vi "TempMeas.vi"() -> ()   [LabVIEW 2017]
uses:
  Control 1.ctl
  <vilib>/DAQmx/read.llb/DAQmx Read (Analog 1D Wfm NChan 1Samp).vi
  <vilib>/DAQmx/miscellaneous.llb/DAQmx Fill In Error Info.vi
panel:
  out "Ścieżka zapisu":path
  out "Waveform Chart - Dark":waveform(dbl)[](graph)
  in  "Refresh Square":bool
  in  "Save Square":bool
  in  "Pause Square":bool
  in  "Start Square":bool
  in  "wybor wykresu":T1
  in  "stop":bool
  out "wsk startu":bool
  in  "Enum":T2(ring)
  in  "DAQmx Task Name":refnum<k21>="temperature_task"
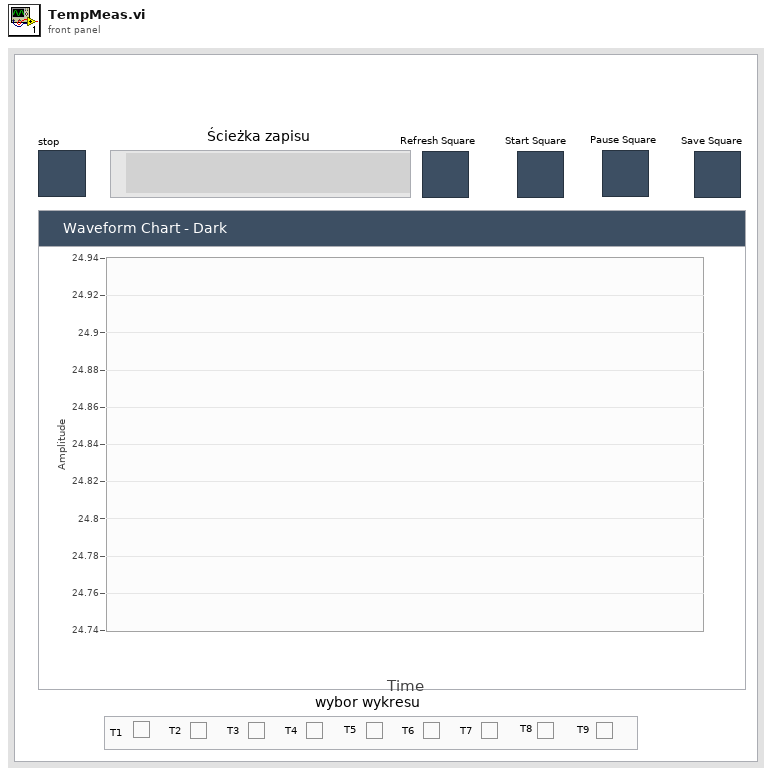
[diagram p1: front panel]
types:
  T1 = typedef "Control 1.ctl" = cluster{"T1":bool, "T2":bool, "T3":bool, "T4":bool, "T6":bool, "T5":bool, "T7":bool, "T8":bool, "T9":bool}
  T2 = enum16{"init", "start", "pause", "save", "exit", "refresh", "wait for event"}
  T3 = enum8{"Enabled", "Disabled", "Disabled and Grayed Out"}
  T4 = enum16{"open", "open or create", "create or replace", "create", "open (read-only)"}
  T5 = enum16{"init", "start", "pause", "save", "exit", "refresh"}
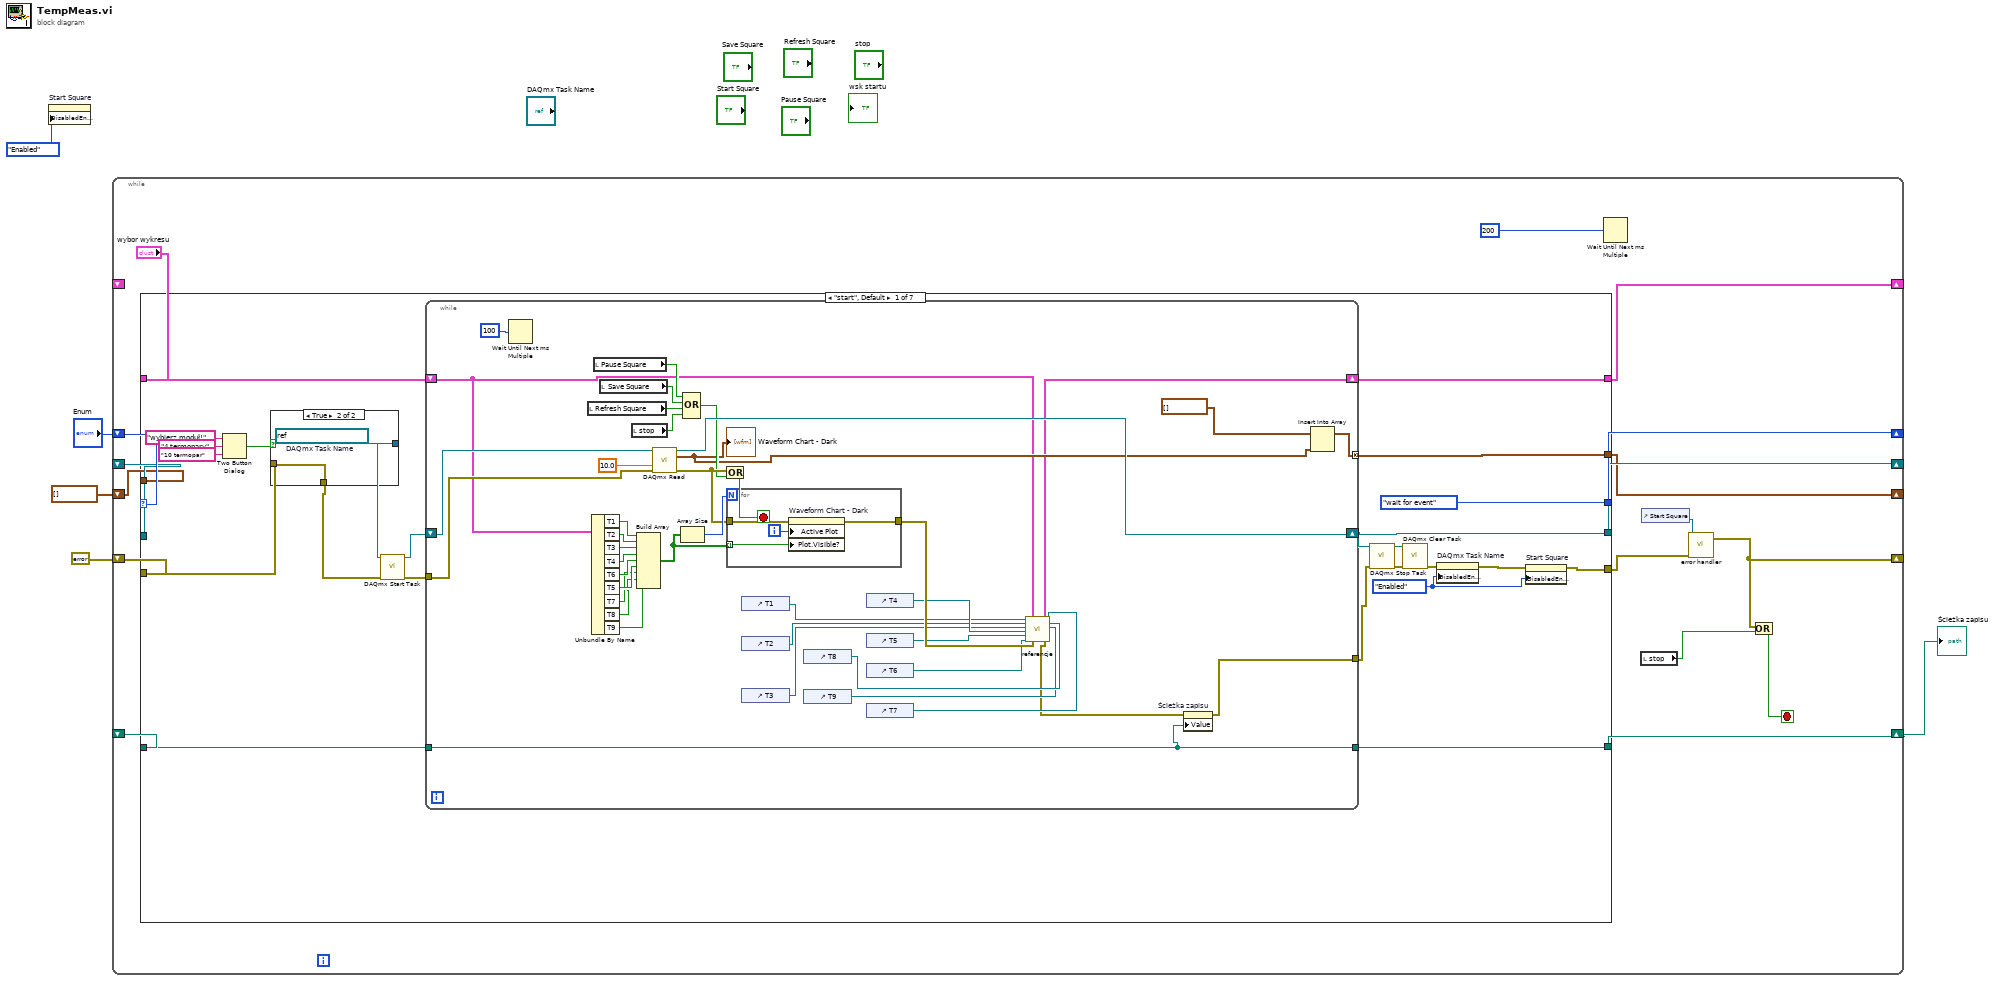
[diagram p0: block diagram]
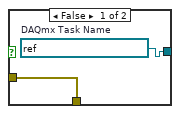
[diagram p2: hidden frame]
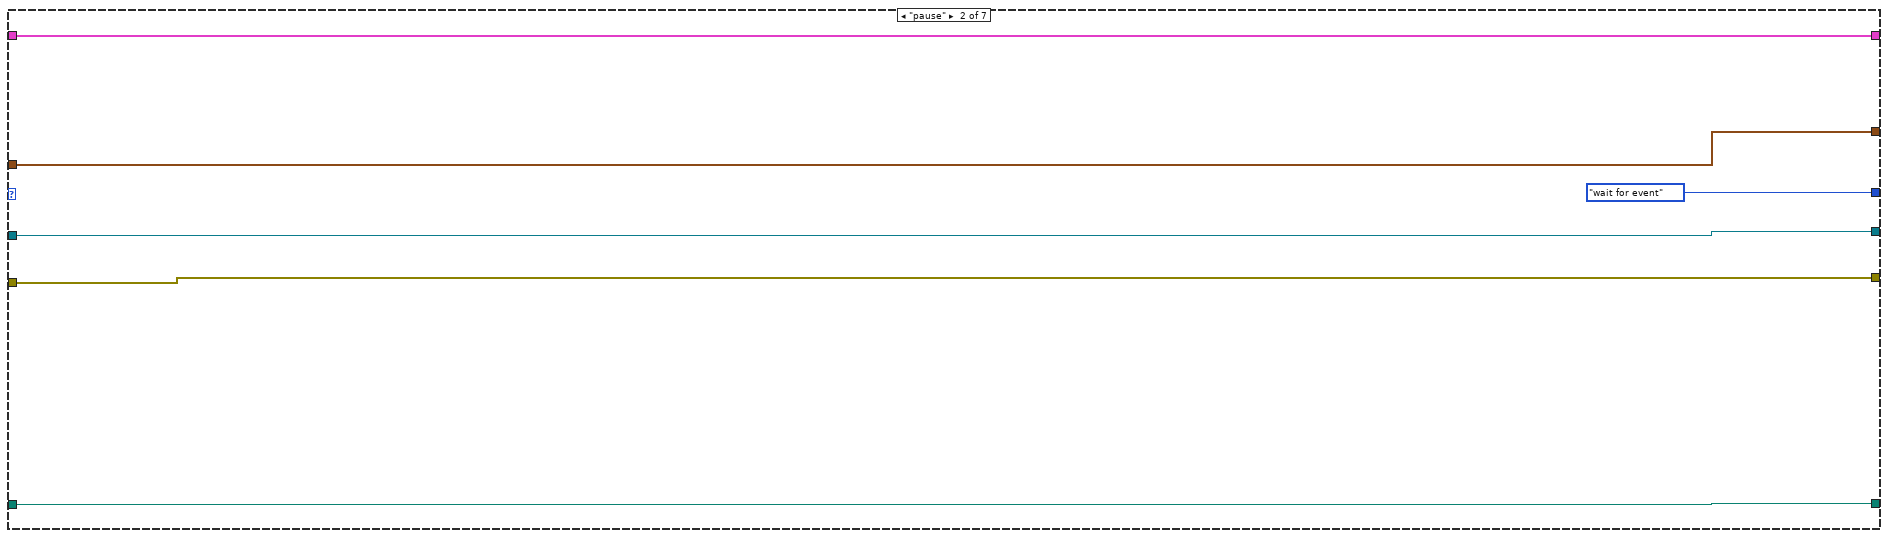
[diagram p3: hidden frame]
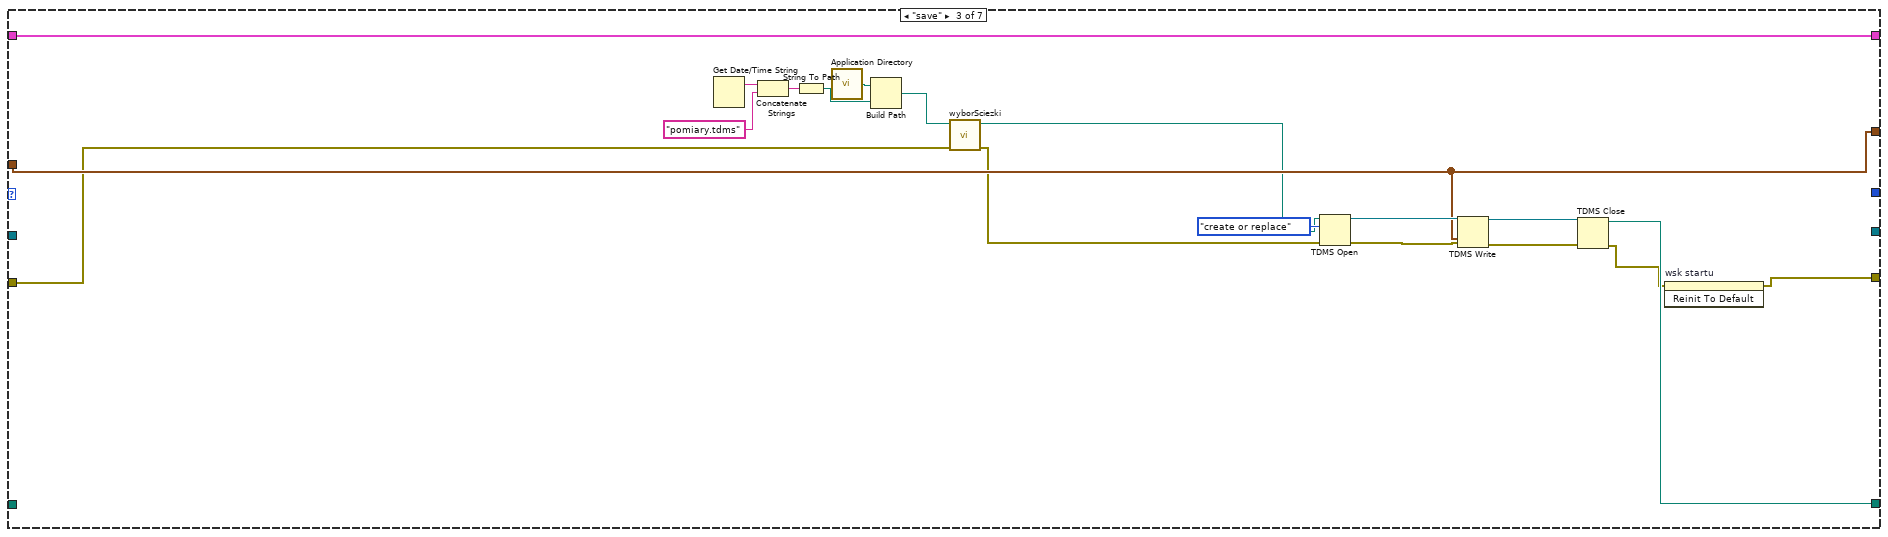
[diagram p4: hidden frame]
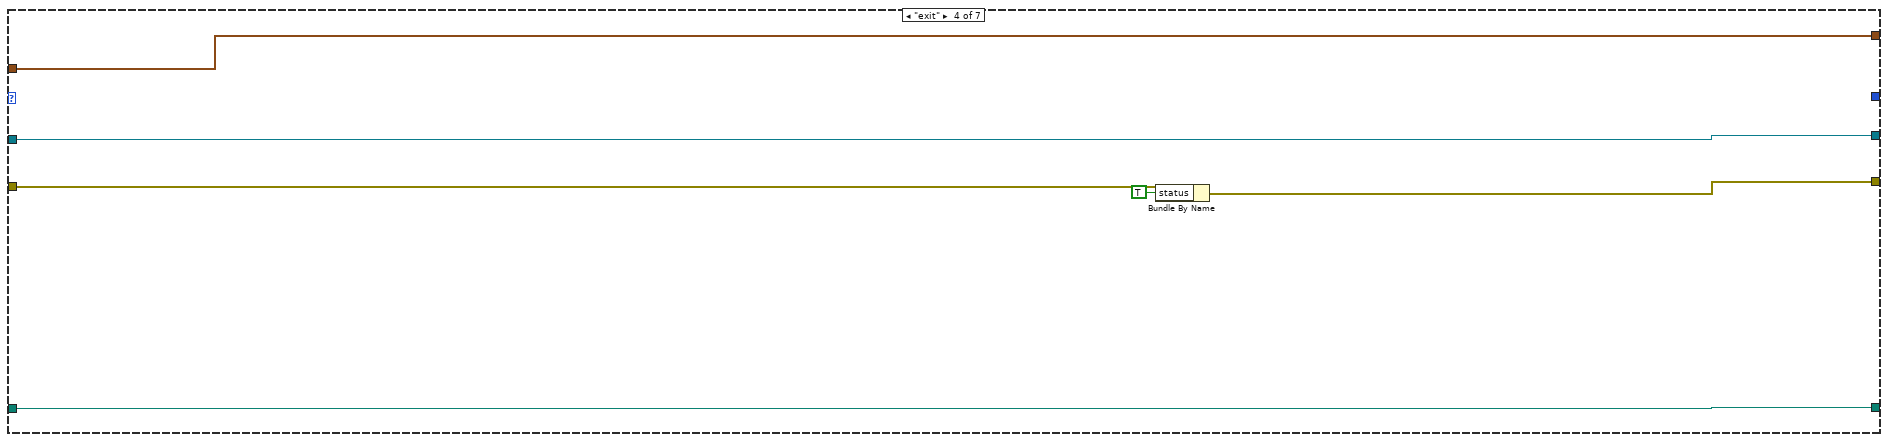
[diagram p5: hidden frame]
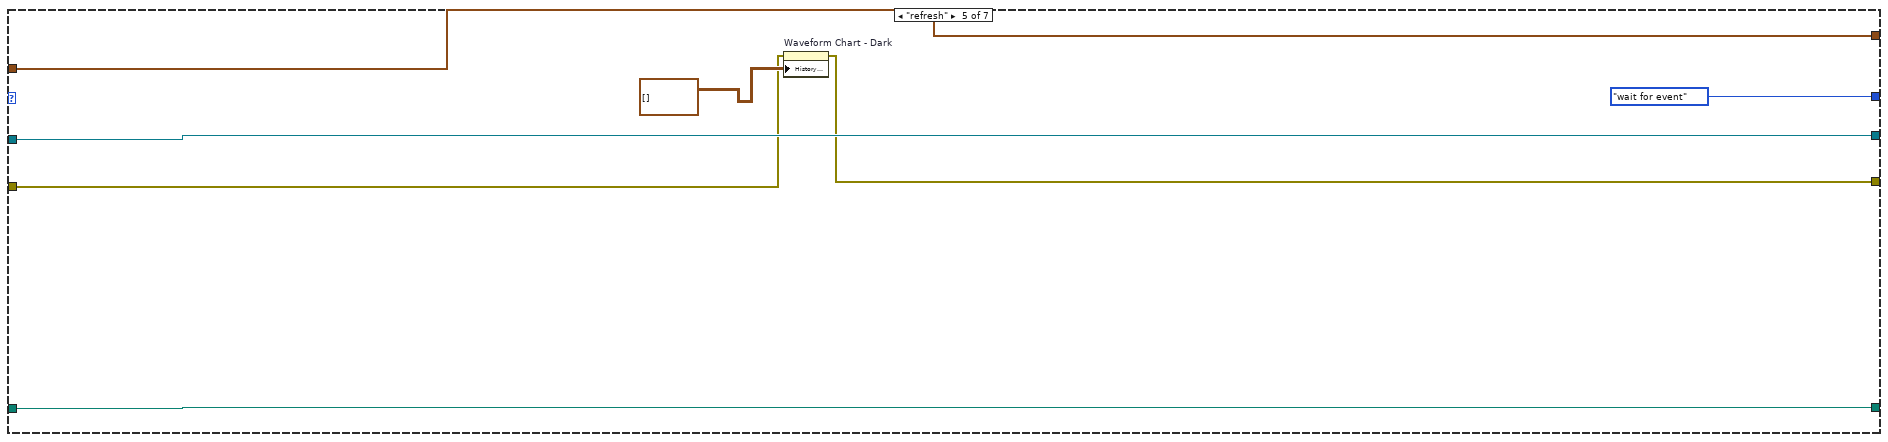
[diagram p6: hidden frame]
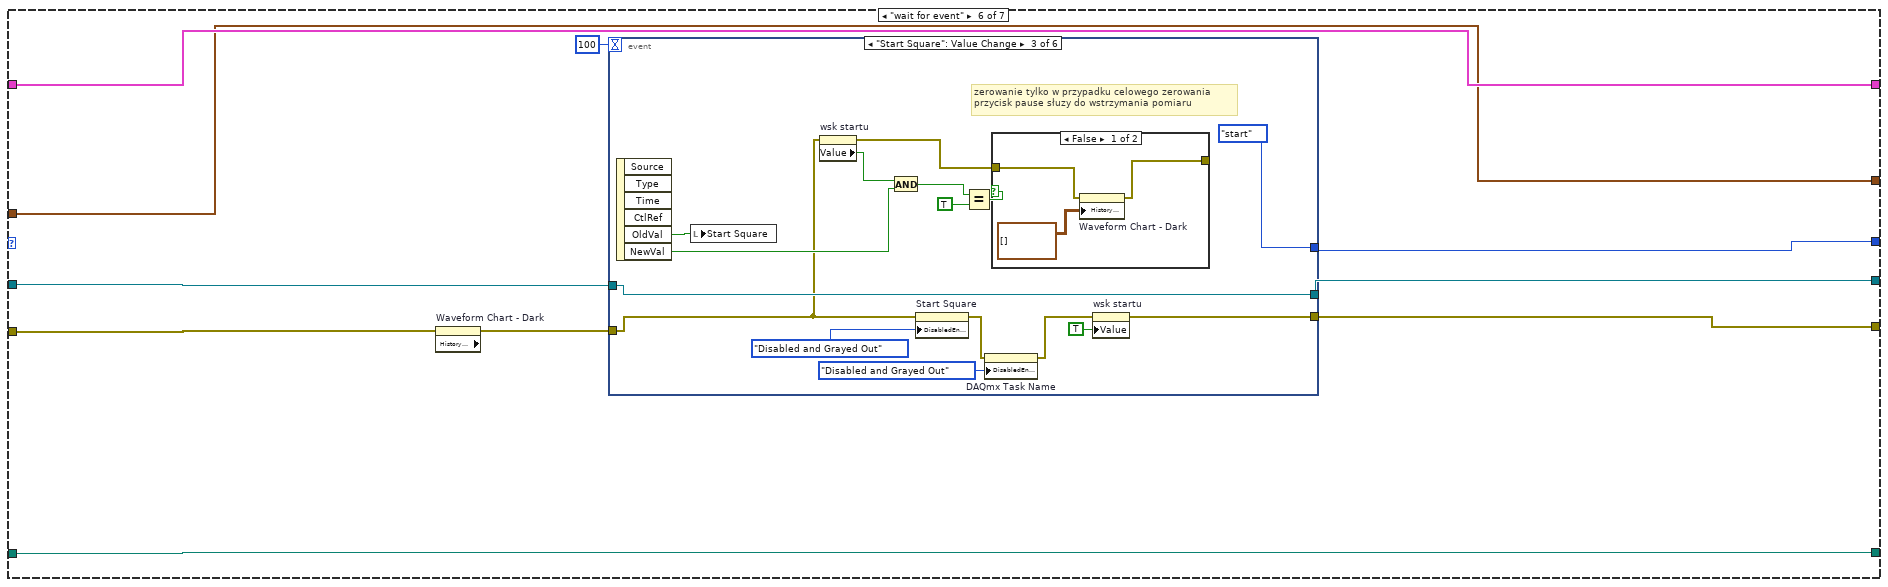
[diagram p7: hidden frame]
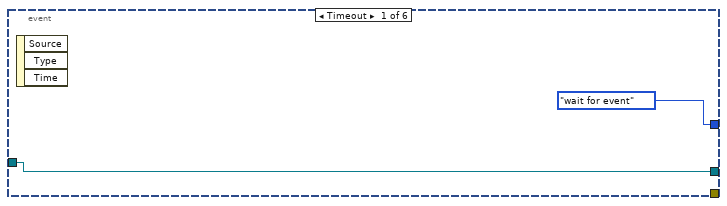
[diagram p8: hidden frame]
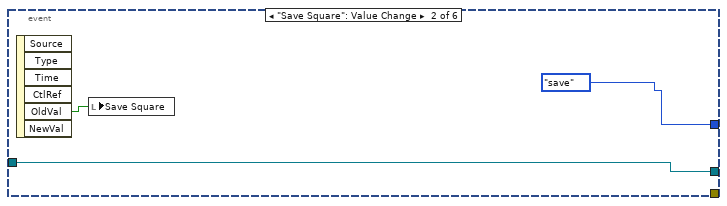
[diagram p9: hidden frame]
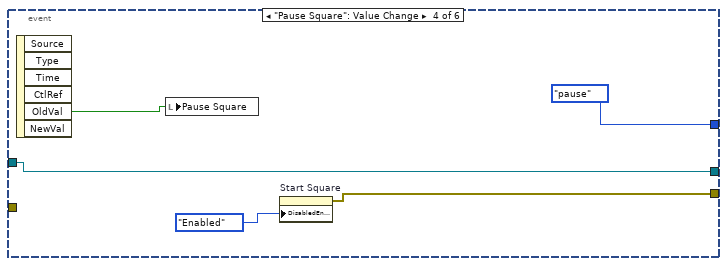
[diagram p11: hidden frame]
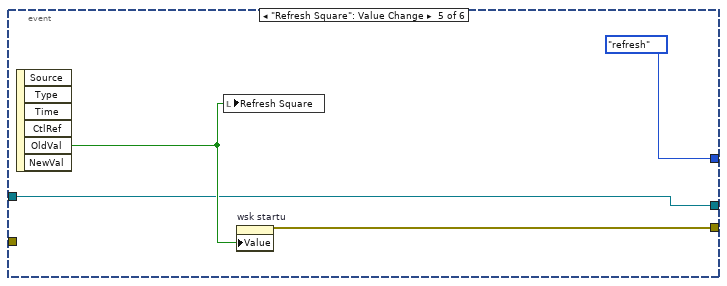
[diagram p12: hidden frame]
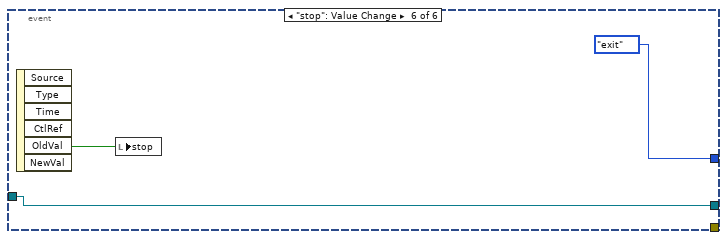
[diagram p13: hidden frame]
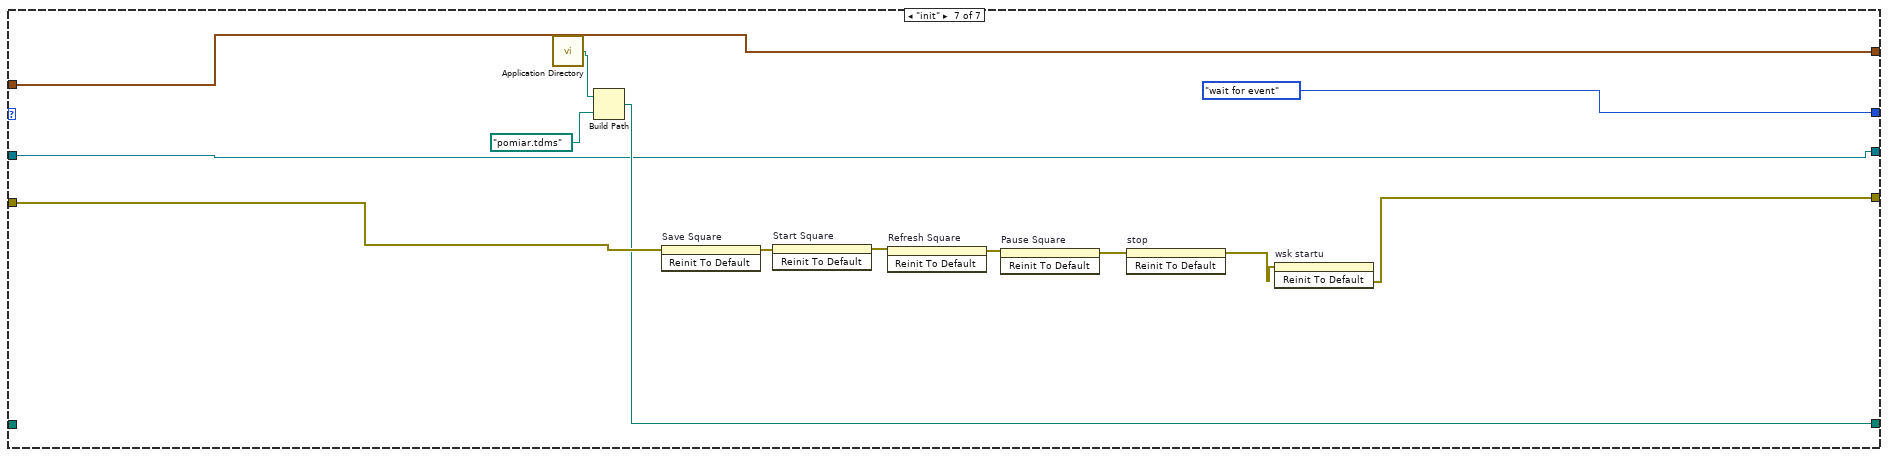
[diagram p14: hidden frame]
diagram:
  n1 = property on="Start Square" class="Bool (strict)"("DisabledEnum"=T3."Enabled" ("Disabled")) -> ()  [unwired: 2 in, 2 out]
  n2 = while {
    shift-right: [w21] -> _
    shift-left: "Enum" -> [w22]
    shift-right: [w9] -> _
    shift-left: errorcluster {"status"=FALSE, "code"=0, "source"=""} ("error constant") -> [w18]
    shift-right: [w7] -> _
    shift-left: _ -> [_]
    shift-right: [w16] -> _
    shift-left: _ -> [w17]
    shift-right: [w12] -> w1
    shift-left: _ -> [w13]
    shift-right: [w11] -> _
    shift-left: waveform(dbl)[] [] ("array") -> [w6]
    stop <- w19 stop-if-true
    n3 = case shown="\"start\", Default" w22 {
      tunnel: [T2."wait for event" ("Enum") T2."wait for event" ("Enum") _ _ T2."wait for event" ("Enum") w142 T2."wait for event" ("Enum")] -> w21
      tunnel: w18 -> [w28 w99 w105 w125 w129 w136 w187]
      tunnel: [w37 w99 w102 w123 w128 w139 w185] -> w10
      tunnel: w17 -> [_ w98 _ w120 w132 w138 w180]
      tunnel: [w43 w97 w119 _ _ w140 _] -> w7
      tunnel: [w42 w98 _ w120 w132 w137 w180] -> w16
      tunnel: "wybor wykresu" -> [w40 w97 w119 _ _ w140 _]
      tunnel: w13 -> [w36 w96 _ w122 w127 w134 _]
      tunnel: [w35 w96 w113 w122 w127 w134 w182] -> w12
      tunnel: [w34 w95 w112 w121 w126 w133 w181] -> w11
      tunnel: w6 -> [_ w95 w112 w121 w126 w133 w181]
      frame "start", Default {
        w31 = T3."Enabled" ("Disabled")
        n4 = Two Button Dialog(message="wybierz moduł!", 1:"10 termopar" ("F button name (\"Cancel\")"), 2:"4 termopary" ("T button name (\"OK\")")) -> (T button?=w29:bool)
        n5 = case shown="True" w29 {
          tunnel: [w47 w49] -> w27
          tunnel: w28 -> [w47 w49]
          tunnel: [w46 w48] -> w26
          frame False {
            w46 = refnum<k21> "Temp_duzy_modul"  # DAQmx Task Name
          }
          frame True {
            w48 = refnum<k21> "temperature_task"  # DAQmx Task Name
          }
        }
        n6 = call <vilib>:"DAQmx Start Task.vi"("task/channels in"=w26, "error in"=w27) -> ("task out"=w41:refnum<k21>, "error out"=w38:errorcluster)  [unwired: 12 in]
        n7 = while {
          shift-right: [w84] -> w42
          shift-left: w41 -> [w90]
          shift-right: [w63] -> w43
          shift-left: w40 -> [w62]
          tunnel: w38 -> [w70]
          tunnel: w36 -> [w50]
          tunnel: [w50] -> w35
          tunnel: [w72] -> w34 mode=concatenating
          tunnel: [w51] -> w30
          stop <- w76 stop-if-true
          n8 = Wait Until Next ms Multiple(millisecond multiple=u32 100) -> ()  [unwired: 1 out]
          n9 = local read "Refresh Square"() -> (w79:bool)
          n10 = Unbundle By Name(w62) -> ("T1"=w87:bool, "T2"=w86:bool, "T3"=w74:bool, "T4"=w85:bool, "T6"=w69:bool, "T5"=w68:bool, "T7"=w67:bool, "T8"=w66:bool, "T9"=w65:bool)
          n11 = local read "Pause Square"() -> (w81:bool)
          n12 = local read "Save Square"() -> (w80:bool)
          n13 = local read "stop"() -> (w78:bool)
          n14 = Build Array(w87, w86, w74, w85, w69, w68, w67, w66, w65) -> (w83:bool[])
          n15 = call-poly <vilib>:"DAQmx Read.vi"("task/channels in"=w90, "timeout"=10.0, "error in"=w70) -> ("task out"=w84:refnum<k21>, "data"=w73:waveform(dbl)[], "error out"=w77:errorcluster)  [unwired: 10 in]
          "Waveform Chart - Dark" <- w73
          n16 = Array Size(array=w83) -> (size(s)=w82:i32)
          n17 = Compound Arithmetic op=OR(w81, w80, w79, w78) -> (w75:bool)
          n18 = Or(x=w77, y=w75) -> (x .or. y?=w76:bool)
          n19 = for {
            N: w82 -> [_]
            tunnel: w83 -> [w91] mode=indexing
            tunnel: w77 -> [w93]
            tunnel: [w92] -> w64
            i -> [w94]
            n20 = property on="Waveform Chart - Dark" class="WFChart (strict)"(error in=w93, "Active Plot"=w94, "Plot.Visible?"=w91) -> (error out=w92:errorcluster)  [unwired: 1 in, 1 out]
          }
          n21 = control-ref of="T1"() -> (w53:refnum<vi>)
          n22 = control-ref of="T2"() -> (w54:refnum<vi>)
          n23 = control-ref of="T3"() -> (w55:refnum<vi>)
          n24 = control-ref of="T8"() -> (w60:refnum<vi>)
          n25 = control-ref of="T9"() -> (w59:refnum<vi>)
          n26 = control-ref of="T4"() -> (w56:refnum<vi>)
          n27 = control-ref of="T5"() -> (w57:refnum<vi>)
          n28 = control-ref of="T6"() -> (w58:refnum<vi>)
          n29 = control-ref of="T7"() -> (w61:refnum<vi>)
          n30 = call "referencje.vi"("T1"=w53, "T2"=w54, "T3"=w55, "T4"=w56, "T5"=w57, "T6"=w58, "wybor wykresu"=w62, "error in (no error)"=w64, "T7"=w61, "T8"=w60, "T9"=w59) -> ("wybor wykresu 2"=w63:T1, "error out"=w52:errorcluster)  [unwired: 7 in]
          n31 = property on="Ścieżka zapisu" class="Path"(error in=w52, "Value"=w50) -> (error out=w51:errorcluster)  [unwired: 1 in, 1 out]
          n32 = Insert Into Array(array=waveform(dbl)[] [], new element=w73) -> (w72:waveform(dbl)[])  [unwired: 1 in]
        }
        n33 = call <vilib>:"DAQmx Stop Task.vi"("task/channels in"=w42, "error in"=w30) -> ("task out"=w45:refnum<k21>, "error out"=w44:errorcluster)  [unwired: 12 in]
        n34 = call <vilib>:"DAQmx Clear Task.vi"("task in"=w45, "error in"=w44) -> ("error out"=w33:errorcluster)  [unwired: 13 in]
        n35 = property on="DAQmx Task Name" class="DAQmxName (strict)"(error in=w33, "DisabledEnum"=w31) -> (error out=w32:errorcluster)  [unwired: 1 in, 1 out]
        n36 = property on="Start Square" class="Bool (strict)"(error in=w32, "DisabledEnum"=w31) -> (error out=w37:errorcluster)  [unwired: 1 in, 1 out]
      }
      frame "pause" {
      }
      frame "save" {
        n37 = Get Date/Time String() -> (date string=w107:string)  [unwired: 3 in, 1 out]
        n38 = Concatenate Strings(w107, "pomiary.tdms" ("name or relative path")) -> (w109:string)
        n39 = String To Path(string=w109) -> (path=w108:path)
        n40 = call <vilib>:"Application Directory.vi"() -> ("Application Directory"=w111:path)
        n41 = Build Path(base path=w111, name or relative path=w108) -> (appended path=w106:path)
        n42 = call "wyborSciezki.vi"("error in (no error)"=w105, "Path Control"=w106) -> ("error out"=w101:errorcluster, "Path Indicator"=w104:path)  [unwired: 6 in]
        n43 = TDMS Open(8:w101, 10:T4."create or replace" ("operation (0:open)"), 11:w104) -> (0:w117:errorcluster, 3:w116:refnum<k34>)  [unwired: 4 in]
        n44 = TDMS Write(0:w116, 9:w112, 11:w117) -> (4:w114:refnum<k34>, 15:w115:errorcluster)  [unwired: 3 in, 2 out]
        n45 = TDMS Close(8:w115, 11:w114) -> (0:w103:errorcluster, 3:w113:path)
        n46 = invoke on="wsk startu" class="Bool (strict)" method="Reinit To Default"(error in=w103) -> (error out=w102:errorcluster)  [unwired: 2 in, 2 out]
      }
      frame "exit" {
        n47 = Bundle By Name(cluster=w125, "status"=TRUE) -> (w123:errorcluster)
      }
      frame "refresh" {
        n48 = property on="Waveform Chart - Dark" class="WFChart (strict)"(error in=w129, "History Data"=waveform(dbl)[][] []) -> (error out=w128:errorcluster)  [unwired: 1 in, 1 out]
      }
      frame "wait for event" {
        n49 = property on="Waveform Chart - Dark" class="WFChart (strict)" props=["History Data"](error in=w136) -> (error out=w135:errorcluster)  [unwired: 1 in, 2 out]
        n50 = event shown="[2] \"Start Square\": Value Change" {
          selector: _ -> [_ _ _ _ _ _]
          dyn-events: _ -> [_ _ _ _ _ _]
          timeout: 100 -> [_ _ _ _ _ _]
          tunnel: [T2."wait for event" ("Enum") T2."save" ("Enum") T5."start" ("Enum") T5."pause" ("Enum") T5."refresh" ("Enum") T5."exit" ("Enum")] -> w142
          tunnel: [_ _ w159 w168 w174 _] -> w139
          tunnel: w138 -> [w144 w146 w161 w170 w173 w177]
          tunnel: [w144 w146 w161 w170 w173 w177] -> w137
          tunnel: w135 -> [_ _ w151 _ _ _]
          event Timeout {
            n51 = event-data() -> ()  [unwired: 1 in, 3 out]
          }
          event "Save Square": Value Change {
            n52 = event-data() -> ("OldVal"=w147:bool)  [unwired: 1 in, 5 out]
            n53 = local write "Save Square"(w147) -> ()
          }
          event "Start Square": Value Change {
            # "zerowanie tylko w przypadku celowego zerowania\nprzycisk pause słuzy do wstrzymania pomiaru"
            n54 = event-data() -> ("OldVal"=w163:bool, "NewVal"=w157:bool)  [unwired: 1 in, 4 out]
            n55 = local write "Start Square"(w163) -> ()
            n56 = property on="wsk startu" class="Bool (strict)"(error in=w151) -> (error out=w152:errorcluster, "Value"=w156:bool)  [unwired: 1 in, 1 out]
            n57 = And(x=w156, y=w157) -> (x .and. y?=w155:bool)
            n58 = property on="Start Square" class="Bool (strict)"(error in=w151, "DisabledEnum"=T3."Disabled and Grayed Out" ("Disabled")) -> (error out=w149:errorcluster)  [unwired: 1 in, 1 out]
            n59 = Equal?(x=w155, y=TRUE) -> (x = y?=w153:bool)
            n60 = property on="DAQmx Task Name" class="DAQmxName (strict)"(error in=w149, "DisabledEnum"=T3."Disabled and Grayed Out" ("Disabled")) -> (error out=w148:errorcluster)  [unwired: 1 in, 1 out]
            n61 = case shown="False" w153 {
              tunnel: w152 -> [w166 w167]
              tunnel: [w164 w167] -> _
              frame False {
                n62 = property on="Waveform Chart - Dark" class="WFChart (strict)"(error in=w166, "History Data"=waveform(dbl)[][] []) -> (error out=w164:errorcluster)  [unwired: 1 in, 1 out]
              }
              frame True {
              }
            }
            n63 = property on="wsk startu" class="Bool (strict)"(error in=w148, "Value"=TRUE ("wsk startu")) -> (error out=w159:errorcluster)  [unwired: 1 in, 1 out]
          }
          event "Pause Square": Value Change {
            n64 = event-data() -> ("OldVal"=w172:bool)  [unwired: 1 in, 5 out]
            n65 = local write "Pause Square"(w172) -> ()
            n66 = property on="Start Square" class="Bool (strict)"("DisabledEnum"=T3."Enabled" ("Disabled")) -> (error out=w168:errorcluster)  [unwired: 2 in, 1 out]
          }
          event "Refresh Square": Value Change {
            n67 = event-data() -> ("OldVal"=w175:bool)  [unwired: 1 in, 5 out]
            n68 = local write "Refresh Square"(w175) -> ()
            n69 = property on="wsk startu" class="Bool (strict)"("Value"=w175) -> (error out=w174:errorcluster)  [unwired: 2 in, 1 out]
          }
          event "stop": Value Change {
            n70 = event-data() -> ("OldVal"=w179:bool)  [unwired: 1 in, 5 out]
            n71 = local write "stop"(w179) -> ()
          }
        }
      }
      frame "init" {
        n72 = call <vilib>:"Application Directory.vi"() -> ("Application Directory"=w184:path)
        n73 = Build Path(base path=w184, name or relative path=path "pomiar.tdms") -> (appended path=w182:path)
        n74 = invoke on="Save Square" class="Bool (strict)" method="Reinit To Default"(error in=w187) -> (error out=w192:errorcluster)  [unwired: 2 in, 2 out]
        n75 = invoke on="Start Square" class="Bool (strict)" method="Reinit To Default"(error in=w192) -> (error out=w190:errorcluster)  [unwired: 2 in, 2 out]
        n76 = invoke on="Refresh Square" class="Bool (strict)" method="Reinit To Default"(error in=w190) -> (error out=w191:errorcluster)  [unwired: 2 in, 2 out]
        n77 = invoke on="Pause Square" class="Bool (strict)" method="Reinit To Default"(error in=w191) -> (error out=w189:errorcluster)  [unwired: 2 in, 2 out]
        n78 = invoke on="stop" class="Bool (strict)" method="Reinit To Default"(error in=w189) -> (error out=w186:errorcluster)  [unwired: 2 in, 2 out]
        n79 = invoke on="wsk startu" class="Bool (strict)" method="Reinit To Default"(error in=w186) -> (error out=w185:errorcluster)  [unwired: 2 in, 2 out]
      }
    }
    n80 = Wait Until Next ms Multiple(millisecond multiple=u32 200) -> ()  [unwired: 1 out]
    n81 = local read "stop"() -> (w20:bool)
    n82 = control-ref of="Start Square"() -> (w8:refnum<vi>)
    n83 = call "error handler.vi"("error in (no error)"=w10, "Boolean in"=w8) -> ("error out"=w9:errorcluster)  [unwired: 9 in]
    n84 = Or(x=w9, y=w20) -> (x .or. y?=w19:bool)
  }
  "Ścieżka zapisu" <- w1
